vi "Auto 1.vi"(8 "Error In":errorcluster) -> (0 "Error Out":errorcluster)   [LabVIEW 2014]
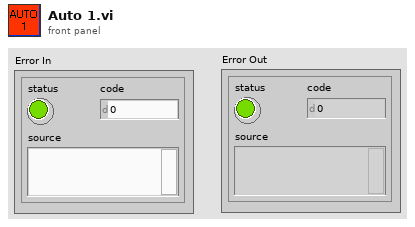
[diagram p1: front panel]
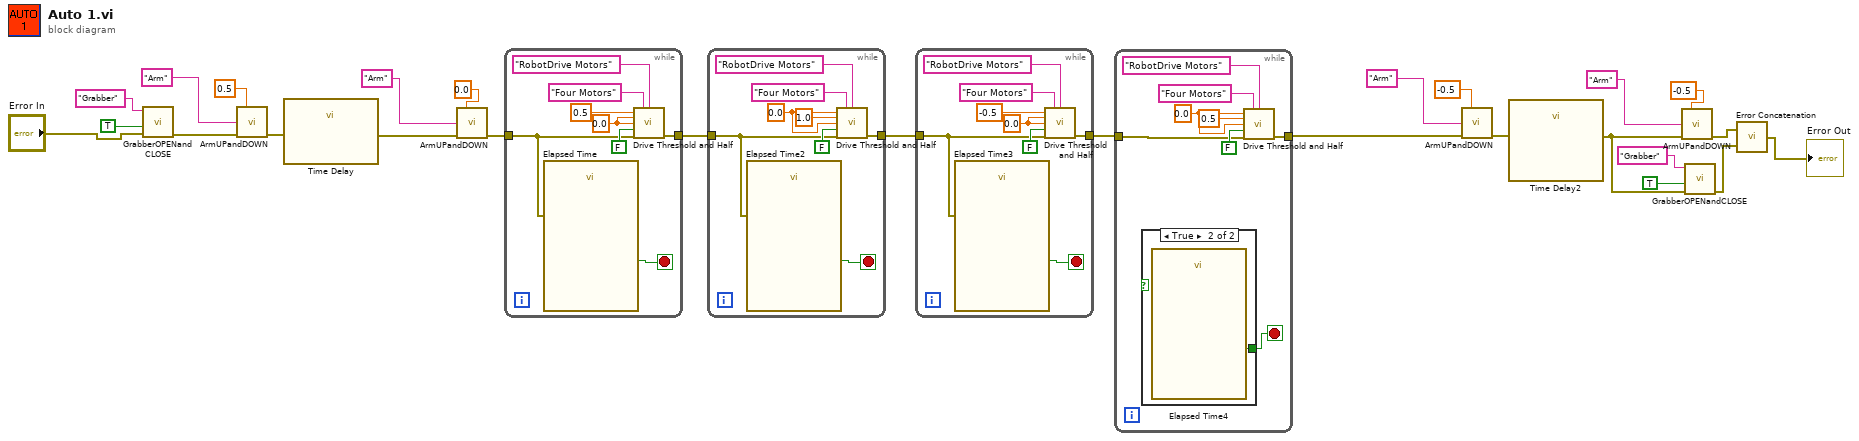
[diagram p0: block diagram]
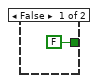
[diagram p2: hidden frame]
diagram:
  n1 = call "GrabberOPENandCLOSE.vi"("Error In"="Error In", "Grabber Open/Close"=TRUE, "refnum name"="Grabber") -> ("Error Out"=w6:errorcluster)  [unwired: 8 in]
  n2 = call "ArmUPandDOWN.vi"("Arm Value"=0.5, "Arm"="Arm" ("refnum name"), "Error In"=w6) -> ("Error Out"=w8:errorcluster)  [unwired: 12 in]
  n3 = call "Time Delay"("error in (no error)"=w8) -> ("error out"=w11:errorcluster)  [unwired: 10 in]
  n4 = call "ArmUPandDOWN.vi"("Arm Value"=0.0, "Arm"="Arm" ("refnum name"), "Error In"=w11) -> ("Error Out"=w13:errorcluster)  [unwired: 12 in]
  n5 = while {
    tunnel: w13 -> [w28]
    tunnel: [w27] -> w12
    stop <- w29 stop-if-true
    w31 = 0.0 ("Arm Value")
    n6 = call "Elapsed Time"("error in (no error)"=w28) -> ("Time has Elapsed"=w29:bool)  [unwired: 11 in, 7 out]
    n7 = call "Drive Threshold and Half.vi"("X In"=0.5, "Drive refnum name"="Four Motors" ("refnum name"), "Send to DB Name"="RobotDrive Motors" ("Name"), "Y In"=w31, "R In"=w31, "Speed Toggle"=FALSE ("Grabber Open/Close"), "Error In"=w28) -> ("Error Out"=w27:errorcluster)  [unwired: 8 in]
  }
  n8 = while {
    tunnel: w12 -> [w37]
    tunnel: [w36] -> w14
    stop <- w38 stop-if-true
    w35 = 0.0 ("X In")
    n9 = call "Elapsed Time2"("error in (no error)"=w37) -> ("Time has Elapsed"=w38:bool)  [unwired: 11 in, 7 out]
    n10 = call "Drive Threshold and Half.vi"("X In"=w35, "Drive refnum name"="Four Motors" ("refnum name"), "Send to DB Name"="RobotDrive Motors" ("Name"), "Y In"=1.0 ("Arm Value"), "R In"=w35, "Speed Toggle"=FALSE ("Grabber Open/Close"), "Error In"=w37) -> ("Error Out"=w36:errorcluster)  [unwired: 8 in]
  }
  n11 = while {
    tunnel: w14 -> [w44]
    tunnel: [w43] -> w15
    stop <- w45 stop-if-true
    w47 = 0.0 ("Arm Value")
    n12 = call "Elapsed Time3"("error in (no error)"=w44) -> ("Time has Elapsed"=w45:bool)  [unwired: 11 in, 7 out]
    n13 = call "Drive Threshold and Half.vi"("X In"=-0.5, "Drive refnum name"="Four Motors" ("refnum name"), "Send to DB Name"="RobotDrive Motors" ("Name"), "Y In"=w47, "R In"=w47, "Speed Toggle"=FALSE ("Grabber Open/Close"), "Error In"=w44) -> ("Error Out"=w43:errorcluster)  [unwired: 8 in]
  }
  n14 = while {
    tunnel: w15 -> [w54]
    tunnel: [w53] -> w22
    stop <- w51 stop-if-true
    w52 = 0.0 ("X In")
    n15 = case shown="True" {
      selector: _ -> [_ _]
      tunnel: [FALSE ("Time has Elapsed") w60] -> w51
      frame False {
      }
      frame True {
        n16 = call "Elapsed Time4"() -> ("Time has Elapsed"=w60:bool)  [unwired: 12 in, 7 out]
      }
    }
    n17 = call "Drive Threshold and Half.vi"("X In"=w52, "Drive refnum name"="Four Motors" ("refnum name"), "Send to DB Name"="RobotDrive Motors" ("Name"), "Y In"=0.5 ("Arm Value"), "R In"=w52, "Speed Toggle"=FALSE ("Grabber Open/Close"), "Error In"=w54) -> ("Error Out"=w53:errorcluster)  [unwired: 8 in]
  }
  n18 = call "ArmUPandDOWN.vi"("Arm Value"=-0.5, "Arm"="Arm" ("refnum name"), "Error In"=w22) -> ("Error Out"=w17:errorcluster)  [unwired: 12 in]
  n19 = call "Time Delay2"("error in (no error)"=w17) -> ("error out"=w24:errorcluster)  [unwired: 10 in]
  n20 = call "ArmUPandDOWN.vi"("Arm Value"=-0.5, "Arm"="Arm" ("refnum name"), "Error In"=w24) -> ("Error Out"=w25:errorcluster)  [unwired: 12 in]
  n21 = call "GrabberOPENandCLOSE.vi"("Error In"=w24, "Grabber Open/Close"=TRUE, "refnum name"="Grabber") -> ("Error Out"=w26:errorcluster)  [unwired: 8 in]
  n22 = call "Error Concatenation.vi"("error in (no error) 2"=w26, "error in (no error)"=w25) -> ("error out"=→"Error Out":errorcluster)
